vi "Write Display Order.vi"(8 "error in (no error)":errorcluster, 10 "Display Order":i32, 11 "Item in":refnum<class "Item.lvclass">) -> (0 "error out":errorcluster, 3 "Item out":refnum<class "Item.lvclass">)   [LabVIEW 2020, in "VI Properties Editor.lvlib" / "Item.lvclass"]
doc: "Gets or sets the display order of the item, as it appears in the top-level project, library, or class it was loaded from."
uses:
  Item.lvclass
  Item.lvclass/Item.ctl
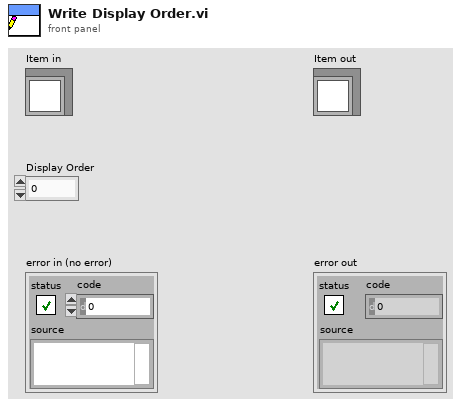
[diagram p1: front panel]
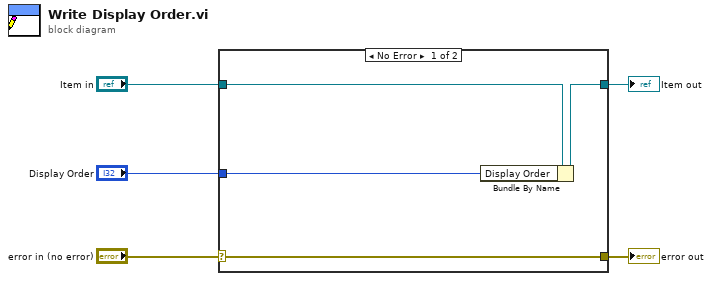
[diagram p0: block diagram]
diagram:
  n1 = case shown="No Error" "error in (no error)" {
    selector: "error in (no error)" -> [w9 w10]
    tunnel: [w9 w10] -> w4
    tunnel: [w7 w11] -> w2
    tunnel: "Item in" -> [w8 w11]
    tunnel: "Display Order" -> [w6 _]
    frame No Error {
      n2 = Bundle By Name(cluster=w8, "Display Order"=w6) -> (w7:refnum<class "Item.lvclass">)
    }
    frame Error {
    }
  }
  "error out" <- w4
  "Item out" <- w2
